vi "gen_termial_data_from_term.vi"(8 "错误输入（无错误）":errorcluster, 10 "type":T1, 11 "Term引用句柄":refnum<vi>) -> (3 "terminal":T2)   [LabVIEW 2020]
uses:
  terminalData.ctl
  terminal_type.ctl
  terminal_direction.ctl
  <vilib>/Utility/Data Type/NI_Data Type.lvlib
panel:
  out "源？":bool
  # "tunnel/judge/shift?"
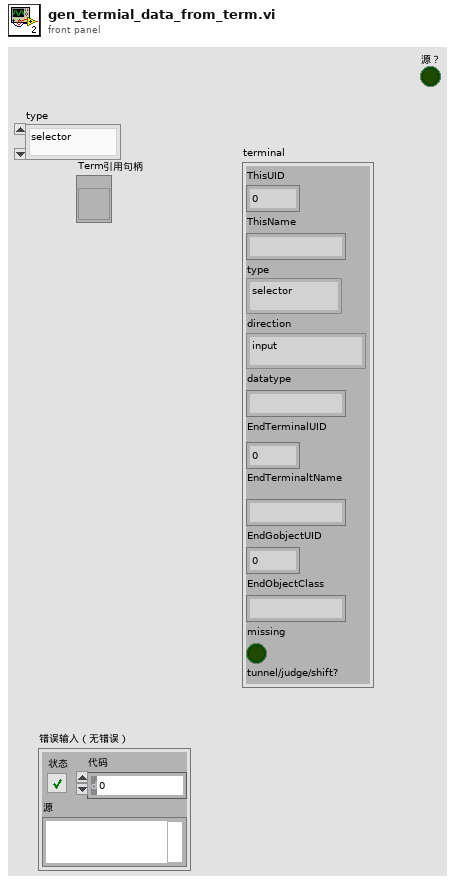
[diagram p1: front panel]
types:
  T1 = typedef "terminal_type.ctl" = enum16{"selector", "tunnel", "shift", "timeout", "normal", "floating"}
  T2 = typedef "terminalData.ctl" = cluster{"ThisUID":i32, "ThisName":string, "type":T1, "direction":T3, "datatype":string, "EndTerminalUID":i32, "EndTerminaltName":string, "EndGobjectUID":i32, "EndObjectClass":string, "missing":bool}
  T3 = typedef "terminal_direction.ctl" = enum16{"input", "output"}
  T4 = typedef "NI_Data Type.lvlib/Data Type.ctl" = enum8{"Invalid Type", "Void", "I8", "I16", "I32", "I64", "U8", "U16", "U32", "U64", "Single Float", "Double Float", "Extended Float", "Single Complex", "Double Complex", "Extended Complex", "Enum U8", "Enum U16", "Enum U32", "Enum U64", "Single Float With Unit", "Double Float With Unit", "Extended Float With Unit", "Single Complex with Unit", "Double Complex with Unit", "Extended Complex with Unit", "Boolean", "String", "Path", "Picture", "Tag", "Array", "Cluster", "Variant", "LV Variant", "Waveform", "Timestamp", "Digital Waveform", "Digital Data", "ExpressData", "Refnum", "External Data", "VI", "Poly VI", "LabVIEW Class Instance", "Fixed Point", "Set Collection", "Map Collection"}
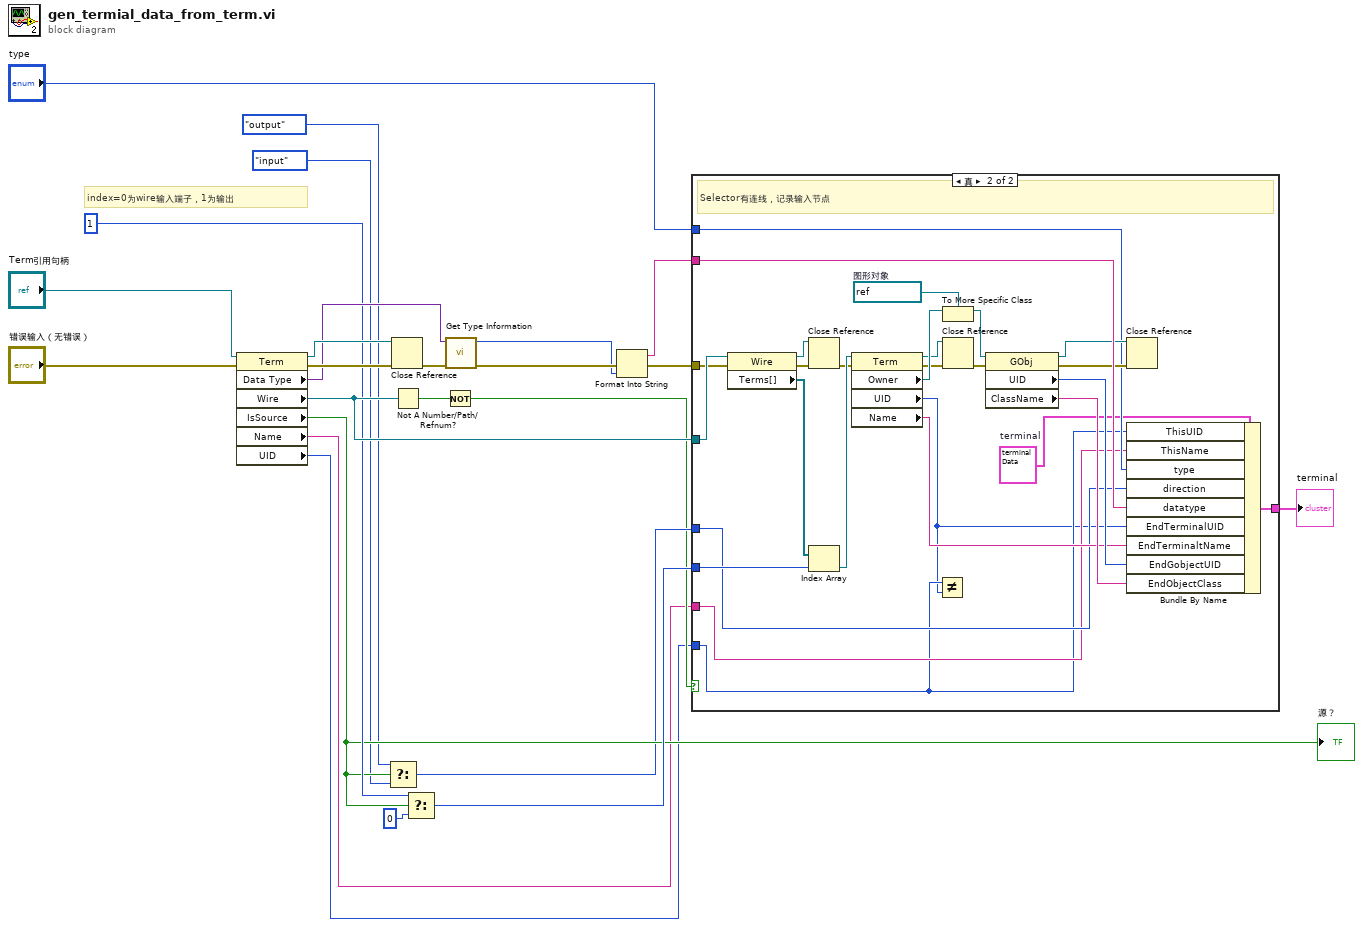
[diagram p0: block diagram]
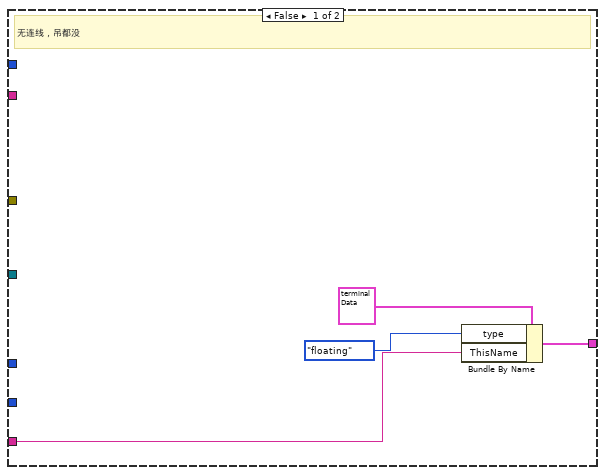
[diagram p2: hidden frame]
diagram:
  # "index=0为wire输入端子，1为输出"
  n1 = property class="Term"(reference="Term引用句柄", error in="错误输入（无错误）") -> (reference out=w15:refnum<vi>, error out=w16:errorcluster, "Data Type"=w13:variant, "Wire"=w21:refnum<vi>, "IsSource"=w9:bool, "Name"=w2:string, "UID"=w1:i32)
  "源？" <- w9
  n2 = Select(t=terminal_direction."output" ("direction"), s=w9, f=terminal_direction."input" ("direction")) -> (s? t:f=w6:T3)
  n3 = Close Reference(reference=w15, error in (no error)=w16) -> (error out=w18:errorcluster)
  n4 = Not A Number/Path/Refnum?(number/path/refnum=w21) -> (NaN/Path/Refnum?=w20:bool)
  n5 = Select(t=1, s=w9, f=0) -> (s? t:f=w10:i32)
  n6 = Not(x=w20) -> (.not. x?=w3:bool)
  n7 = call <vilib>:"Get Type Information.vi"("error in (no error)"=w18, "variant"=w13) -> ("error out"=w19:errorcluster, "type"=w14:T4)  [unwired: 5 in, 3 out]
  n8 = Format Into String(error in=w19, w14) -> (resulting string=w22:string, error out=w23:errorcluster)  [unwired: 2 in]
  n9 = case shown="真" w3 {
    tunnel: w21 -> [_ w55]
    tunnel: w22 -> [_ w49]
    tunnel: w23 -> [_ w37]
    tunnel: [w26 w29] -> w24
    tunnel: w10 -> [_ w36]
    tunnel: w6 -> [_ w35]
    tunnel: "type" -> [_ w34]
    tunnel: w2 -> [w25 w33]
    tunnel: w1 -> [_ w32]
    frame False {
      # "无连线，吊都没"
      n10 = Bundle By Name(cluster=T2 {"ThisUID"=0, "ThisName"="", "type"=enum."selector", "direction"=enum."input", "datatype"="", "EndTerminalUID"=0, "EndTerminaltName"="", "EndGobjectUID"=0, "EndObjectClass"="", "missing"=FALSE} ("terminal 2"), "type"=terminal_type."floating", "ThisName"=w25) -> (w26:T2)
    }
    frame True {
      w30 = T2 {"ThisUID"=0, "ThisName"="", "type"=enum."selector", "direction"=enum."input", "datatype"="", "EndTerminalUID"=0, "EndTerminaltName"="", "EndGobjectUID"=0, "EndObjectClass"="", "missing"=FALSE}  # terminal
      w51 = refnum<vi> refnum  # 图形对象
      # "Selector有连线，记录输入节点"
      n11 = property class="Wire"(reference=w55, error in=w37) -> (reference out=w45:refnum<vi>, error out=w44:errorcluster, "Terms[]"=w54:refnum<vi>[])
      n12 = Close Reference(reference=w45, error in (no error)=w44) -> (error out=w43:errorcluster)
      n13 = Index Array(array=w54, index=w36) -> (element=w53:refnum<vi>)
      n14 = property class="Term"(reference=w53, error in=w43) -> (reference out=w42:refnum<vi>, error out=w41:errorcluster, "Owner"=w52:refnum<vi>, "UID"=w31:i32, "Name"=w46:string)
      n15 = Not Equal?(x=w32, y=w31) -> ()  [unwired: 1 out]
      n16 = To More Specific Class(target class=w51, reference=w52) -> (specific class reference=w50:refnum<vi>)  [unwired: 1 in, 1 out]
      n17 = Close Reference(reference=w42, error in (no error)=w41) -> (error out=w40:errorcluster)
      n18 = property class="GObj"(reference=w50, error in=w40) -> (reference out=w39:refnum<vi>, error out=w38:errorcluster, "UID"=w48:i32, "ClassName"=w47:string)
      n19 = Close Reference(reference=w39, error in (no error)=w38) -> ()  [unwired: 1 out]
      n20 = Bundle By Name(cluster=w30, "ThisUID"=w32, "ThisName"=w33, "type"=w34, "direction"=w35, "datatype"=w49, "EndTerminalUID"=w31, "EndTerminaltName"=w46, "EndGobjectUID"=w48, "EndObjectClass"=w47) -> (w29:T2)
    }
  }
  "terminal" <- w24
